vi "pharosTriggersSave.vi"   [LabVIEW 2017]
uses:
  globalUtilities.vi
types:
  T1 = enum16{"open", "replace", "create", "open or create", "replace or create", "replace or create with confirmation"}
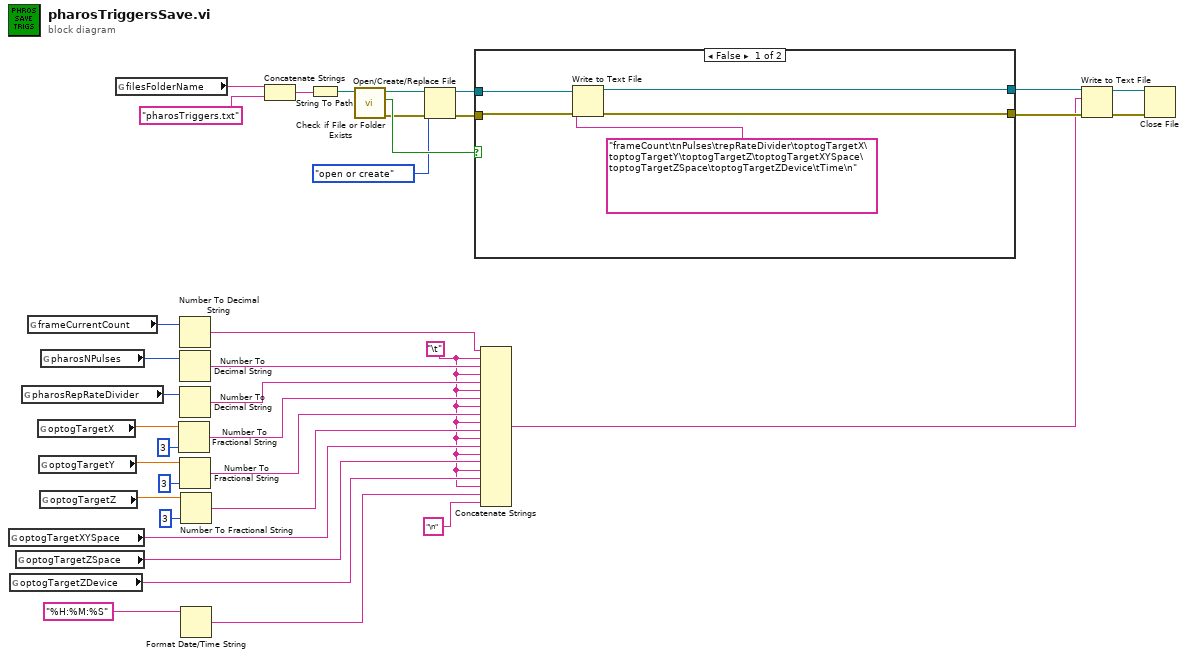
[diagram p0: block diagram]
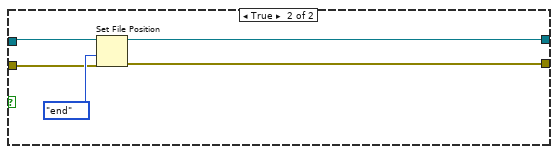
[diagram p2: hidden frame]
diagram:
  w3 = "\t"
  n1 = global read "globalUtilities.vi" "optogTargetXYSpace"() -> (w7:string)
  n2 = global read "globalUtilities.vi" "optogTargetZDevice"() -> (w5:string)
  n3 = global read "globalUtilities.vi" "optogTargetZSpace"() -> (w6:string)
  n4 = global read "globalUtilities.vi" "pharosRepRateDivider"() -> (w21:i32)
  n5 = global read "globalUtilities.vi" "frameCurrentCount"() -> (w23:i32)
  n6 = global read "globalUtilities.vi" "optogTargetX"() -> (w16:dbl)
  n7 = global read "globalUtilities.vi" "optogTargetY"() -> (w12:dbl)
  n8 = global read "globalUtilities.vi" "optogTargetZ"() -> (w10:dbl)
  n9 = global read "globalUtilities.vi" "pharosNPulses"() -> (w22:i32)
  n10 = global read "globalUtilities.vi" "filesFolderName"() -> (w37:string)
  n11 = Number To Fractional String(number=w16, precision (6)=i16 3) -> (F-format string=w14:string)  [unwired: 2 in]
  n12 = Number To Decimal String(number=w23) -> (decimal integer string=w20:string)  [unwired: 1 in]
  n13 = Number To Decimal String(number=w22) -> (decimal integer string=w19:string)  [unwired: 1 in]
  n14 = Number To Decimal String(number=w21) -> (decimal integer string=w18:string)  [unwired: 1 in]
  n15 = Number To Fractional String(number=w12, precision (6)=i16 3) -> (F-format string=w11:string)  [unwired: 2 in]
  n16 = Number To Fractional String(number=w10, precision (6)=i16 3) -> (F-format string=w8:string)  [unwired: 2 in]
  n17 = Format Date/Time String(time format string (%c)="%H:%M:%S") -> (date/time string=w2:string)  [unwired: 2 in]
  n18 = Concatenate Strings(w37, "pharosTriggers.txt" ("string")) -> (w35:string)
  n19 = String To Path(string=w35) -> (path=w34:path)
  n20 = call <vilib>:"Check if File or Folder Exists.vi"("path"=w34) -> ("error out"=w32:errorcluster, "file or folder exists?"=w33:bool, "dup path"=w31:path)  [unwired: 8 in]
  n21 = Open/Create/Replace File(file path (use dialog)=w31, error in=w32, operation (0:open)=T1."open or create") -> (refnum out=w29:refnum<file>, error out=w28:errorcluster)  [unwired: 3 in, 1 out]
  n22 = case shown="False" w33 {
    tunnel: w29 -> [w42 w47]
    tunnel: w28 -> [w41 w45]
    tunnel: [w39 w44] -> w27
    tunnel: [w38 w43] -> w26
    frame False {
      n23 = Write to Text File(file (use dialog)=w42, text="frameCount\tnPulses\trepRateDivider\toptogTargetX\toptogTargetY\toptogTargetZ\toptogTargetXYSpace\toptogTargetZSpace\toptogTargetZDevice\tTime\n", error in=w41) -> (refnum out=w39:refnum<file>, error out=w38:errorcluster)  [unwired: 1 in, 1 out]
    }
    frame True {
      n24 = Set File Position(refnum=w47, from (0:start)=enum16{"start", "end", "current"}."end", error in=w45) -> (refnum out=w44:refnum<file>, error out=w43:errorcluster)  [unwired: 1 in]
    }
  }
  n25 = Concatenate Strings(w20, w3, w19, w3, w18, w3, w14, w3, w11, w3, w8, w3, w7, w3, w6, w3, w5, w3, w2, "\n") -> (w17:string)
  n26 = Write to Text File(file (use dialog)=w27, text=w17, error in=w26) -> (refnum out=w25:refnum<file>, error out=w24:errorcluster)  [unwired: 1 in, 1 out]
  n27 = Close File(refnum=w25, error in=w24) -> ()  [unwired: 2 out]
